vi "Update State.vi"(9 "text":string, 11 "end state in":dbl[](array[numeric])) -> (1 "GCode":cluster{"Command":string, "End State":dbl[]}, 3 "end state out":dbl[](array[numeric]))   [LabVIEW 2024]
uses:
  <vilib>/Utility/error.llb/Trim Whitespace One-Sided.vi
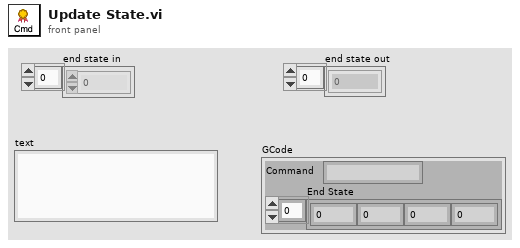
[diagram p1: front panel]
types:
  T1 = cluster{"trimmed string":string, "Array out":dbl[]}
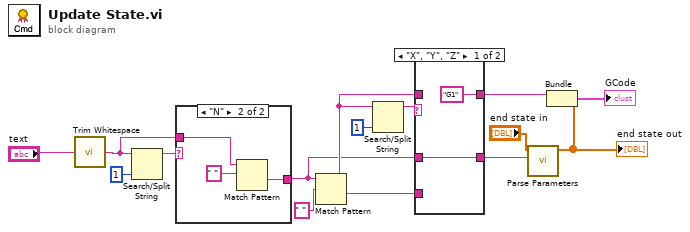
[diagram p0: block diagram]
diagram:
  n1 = call <vilib>:"Trim Whitespace.vi"("string"="text") -> ("trimmed string"=w2:string)  [unwired: 1 in]
  n2 = Search/Split String(string=w2, offset (0)=1) -> (substring before match=w3:string)  [unwired: 1 in, 2 out]
  n3 = case shown="\"N\"" w3 {
    tunnel: w2 -> [w16 w18]
    tunnel: [w16 w17] -> w1
    frame Default {
    }
    frame "N" {
      n4 = Match Pattern(string=w18, regular expression=" ") -> (after substring=w17:string)  [unwired: 1 in, 3 out]
    }
  }
  n5 = Match Pattern(string=w1, regular expression=" ") -> (before substring=w13:string, after substring=w11:string)  [unwired: 1 in, 2 out]
  n6 = Search/Split String(string=w13, offset (0)=1) -> (substring before match=w14:string)  [unwired: 1 in, 2 out]
  n7 = case shown="\"X\", \"Y\", \"Z\"" w14 {
    tunnel: [w21 w23] -> w10
    tunnel: w11 -> [_ w23]
    tunnel: w1 -> [w21 _]
    tunnel: ["G1" ("text") w22] -> w12
    tunnel: w13 -> [_ w22]
    frame "X", "Y", "Z" {
    }
    frame Default {
    }
  }
  n8 = call <userlib>:"Parse Parameters.vi"("String"=w10, "Array in"="end state in") -> ("Array out"=w7:dbl[])  [unwired: 9 in]
  "end state out" <- w7
  n9 = Bundle("trimmed string"=w12, "Array out"=w7) -> (→"GCode":T1)  [unwired: 1 in]
